vi "SHA-2-U64_preprocess_chunk.vi"(8 "error in (no error)":errorcluster, 11 "Chunk in":string) -> (0 "error out":errorcluster, 3 "Processed chunk out":u64[](array[numeric]))   [LabVIEW 2012, in "Encryption.lvlib"]
uses:
  Encryption.lvlib
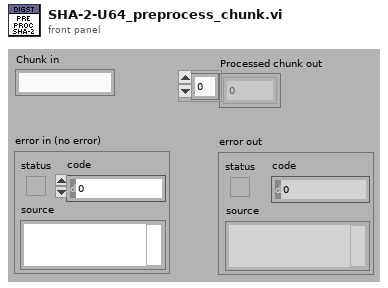
[diagram p1: front panel]
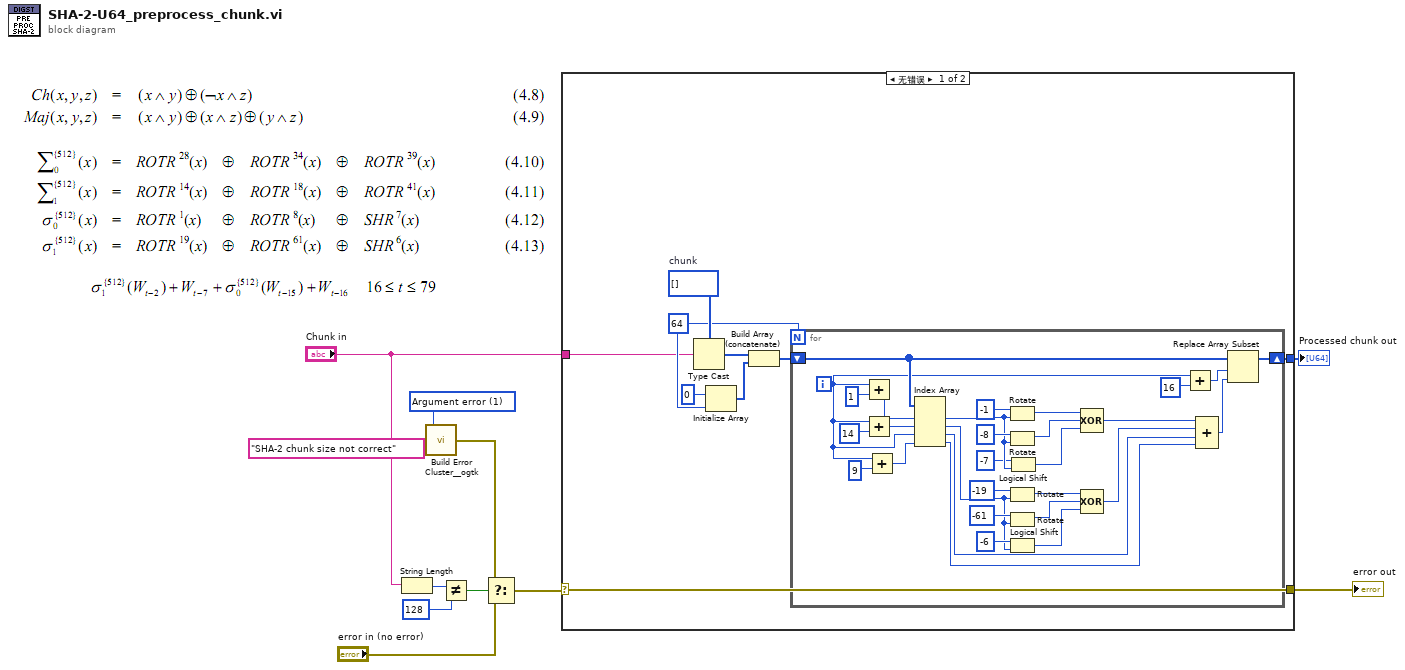
[diagram p0: block diagram]
diagram:
  w5 = 1 items=["No error", "Argument error", "Memory is full", "Out of zone", "End of file", "File already open", "Generic file I/O error", "File not found", "File permission error", "Disk is full", "Duplicate path", "Too many files open", "System feature not enabled", "Resource file not found", "Cannot add resource", "Resource not found", "Image not found", "Image memory error", "Pen does not exist", "Config type invalid", "Config token not found", "Config parse error", "Config memory error", "Bad external code format", "Bad external code offset", "External code not present", "Null window", "Destroy window error", "Null menu", "Print aborted", "Bad print record", "Print driver error", "Windows error during printing", "Memory error during printing", "Print dialog error", "Generic print error", "Invalid device refnum", "Device not found", "Device parameter error", "Device unit error", "Cannot open device", "Device call aborted", "Generic error", "Cancelled by user", "Object ID too low", "Object ID too high", "Object not in heap", "Unknown heap", "Unknown object (invalid DefProc)", "Unknown object (DefProc not in table)", "Message out of range", "Invalid (null) method", "Unknown message", "Manager call not supported", "Bad address", "Network operation in progress", "Network operation timed out", "Connection is busy", "Network attribute not supported", "Network error", "Address in use", "System out of memory", "Connection aborted", "Connection refused", "Not connected", "Already connected", "Connection closed", "Initialization error (interapplication manager)", "Bad occurrence", "Wait on unbound occurrence handler", "Occurrence queue overflow", "Datalog type conflict", "Unused", "Unrecognized type (interapplication manager)", "Memory corrupt", "Failed to make temporary DLL", "Old CIN version", "Drag socket not found", "Failed to load drop-object", "Failed to register OLE object", "Failed to release OLE object", "Format specifier type mismatch", "Unknown format specifier", "Too few format specifiers", "Too many format specifiers", "Scan failed", "Newer CIN version", "Error converting to variant", "Runtime menu error", "Password tampered", "Variant attribute not found", "Incompatible variant data type", "Event data is not available", "Event Store is not present", "Occurrence is not found", "Event Queue is not created", "Event info is not available", "Refnum passed is NULL", "Error retrieving Class GUID", "Error retrieving CoClass GUID", "Error retrieving TypeLib GUID.", "Bad built application magic bytes.", "Specific driver is different from the specific driver associated with the Logical Name.", "There is no session opened to the class driver.", "Max Error", "MAX - Error with config objects", "MAX - Error loading configuration", "MAX - Group not supported"]
  n1 = String Length(string="Chunk in") -> (length=w10:i32)
  n2 = call <userlib>:"Build Error Cluster__ogtk.vi"("String to Prepend to source (\"\")"="SHA-2 chunk size not correct" ("String to Prepend to source (\"\")"), "code"=w5) -> ("error out"=w7:errorcluster)
  n3 = Not Equal?(x=w10, y=128) -> (x != y?=w8:bool)
  n4 = Select(t=w7, s=w8, f="error in (no error)") -> (s? t:f=w3:errorcluster)
  n5 = case shown="无错误" w3 {
    selector: w3 -> [w12 w51]
    tunnel: [w19 _] -> w11
    tunnel: "Chunk in" -> [w13 _]
    tunnel: [w12 w51] -> w1
    frame No Error {
      w20 = u64[] []  # chunk
      w18 = 64 ("dimension size")
      n6 = Type Cast(type=w20, x=w13) -> (*(type *) &x=w15:u64[])
      n7 = Initialize Array(u64 0, w18) -> (w16:u64[])
      n8 = Build Array (concatenate)(w15, w16) -> (w17:u64[])
      n9 = for {
        N: w18 -> [_]
        shift-right: [w45] -> w19
        shift-left: w17 -> [w46]
        i -> [w27]
        n10 = Add(x=w27, y=1 ("value")) -> (x+y=w29:i32)
        n11 = Add(x=w27, y=14 ("value")) -> (x+y=w28:i32)
        n12 = Add(x=w27, y=9 ("value")) -> (x+y=w25:i32)
        n13 = Index Array(array=w46, index #1=w29, index #2=w28, index #3=w27, index #4=w25) -> (element #1=w23:u64, element #2=w31:u64, element #3=w26:u64, element #4=w24:u64)
        n14 = Rotate(1:w23, 2:i8 -1 ("y")) -> (0:w41:u64)
        n15 = Rotate(1:w23, 2:i8 -8 ("y")) -> (0:w40:u64)
        n16 = Rotate(1:w31, 2:i8 -19 ("y")) -> (0:w34:u64)
        n17 = Rotate(1:w31, 2:i8 -61 ("y")) -> (0:w35:u64)
        n18 = Logical Shift(y=i8 -6, x=w31) -> (x << y=w37:u64)
        n19 = Logical Shift(y=i8 -7, x=w23) -> (x << y=w22:u64)
        n20 = Compound Arithmetic op=XOR(w41, w40, w22) -> (w38:u64)
        n21 = Compound Arithmetic op=XOR(w34, w35, w37) -> (w30:u64)
        n22 = Add(x=w27, y=16) -> (x+y=w44:i32)
        n23 = Compound Arithmetic op=ADD(w38, w30, w26, w24) -> (w39:u64)
        n24 = Replace Array Subset(array=w46, new element=w39, index=w44) -> (w45:u64[])
      }
    }
    frame Error {
    }
  }
  "Processed chunk out" <- w11
  "error out" <- w1
